vi "HVBuncher.UpdateChannelVoltage.vi"(0 "i ref in":refnum<vi>, 1 "channel":i32, 2 "ChannelVoltages":dbl[](array[numeric]), 3 "ms timeout (10000)":i32=10000, 5 "error in (no error)":errorcluster) -> (14 "i ref out":refnum<vi>, 16 "actVoltage":dbl, 18 "timed out":bool, 19 "error out":errorcluster)   [LabVIEW 2014, in "HVBuncher.lvlib"]
doc: "Gets the voltage from DIM."
uses:
  HVBuncher.lvlib
  CSCore/CSApplicationBaseClasses/PSChannelBase/PSChannelBase.directionType.ctl
  CSCore/CSApplicationBaseClasses/PSChannelBase/PSChannelBase.serviceType.ctl
  CSlibraries/UtilityLib/UtilityLib.valueStatus.ctl
  CSCore/CSApplicationBaseClasses/PSChannelBase/PSChannelBase.lvlib
  CSlibraries/UtilityLib/UtilityLib.lvlib
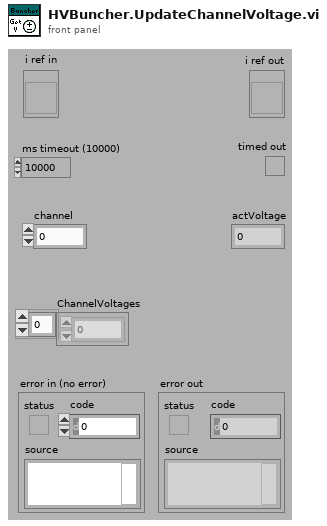
[diagram p1: front panel]
types:
  T1 = typedef "UtilityLib.lvlib/UtilityLib.valueStatus.ctl" = enum16{"no info available", "stand by/off", "on", "warning", "alarm/malfunction", "not implemented", "user action required", "important information", "system default", "control default", "indicator default", "button default"}
  T2 = typedef "PSChannelBase.lvlib/PSChannelBase.serviceType.ctl" = enum16{"onOff", "voltage", "current", "tripCurrent", "rampUpSpeed", "rampDownSpeed", "status"}
  T3 = typedef "PSChannelBase.lvlib/PSChannelBase.directionType.ctl" = enum16{"unknown", "update actual value", "update nominal value", "update both"}
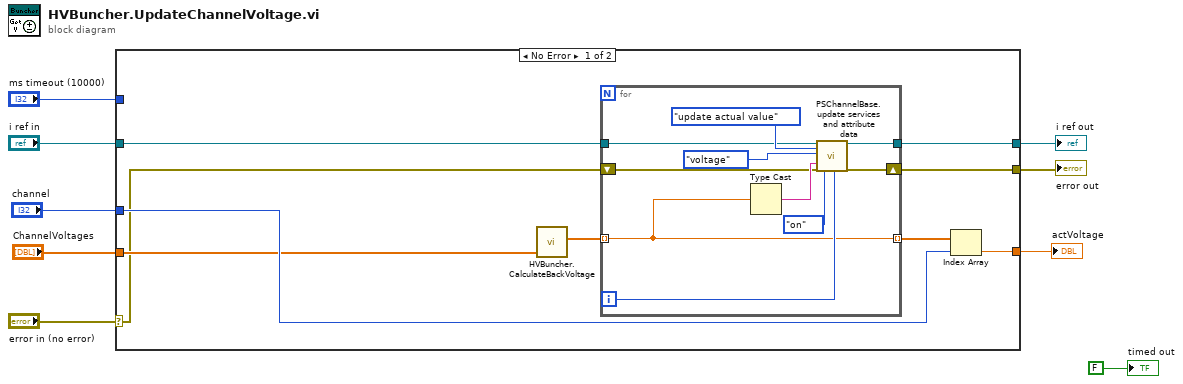
[diagram p0: block diagram]
diagram:
  n1 = case shown="No Error" "error in (no error)" {
    selector: "error in (no error)" -> [w11 w30]
    tunnel: "i ref in" -> [w10 w29]
    tunnel: "ms timeout (10000)" -> [_ _]
    tunnel: "channel" -> [w13 _]
    tunnel: [w15 w30] -> w4
    tunnel: [w16 w29] -> w3
    tunnel: [w17 _] -> w2
    tunnel: "ChannelVoltages" -> [w12 _]
    frame No Error {
      n2 = call "HVBuncher.CalculateBackVoltage.vi"("ChannelVoltages"=w12) -> ("actlVoltages"=w14:dbl[])  [unwired: 10 in]
      n3 = for {
        tunnel: w10 -> [w20]
        shift-right: [w24] -> w15
        shift-left: w11 -> [w21]
        tunnel: [w23] -> w16
        tunnel: [w19] -> w18 mode=indexing
        tunnel: w14 -> [w19] mode=indexing
        i -> [w22]
        n4 = Type Cast(x=w19) -> (*(type *) &x=w26:string)  [unwired: 1 in]
        n5 = call "PSChannelBase.update services and attribute data.vi"("i ref in"=w20, "direction"=PSChannelBase.directionType."update actual value", "service"=PSChannelBase.serviceType."voltage", "value"=w26, "error in (no error)"=w21, "quality"=UtilityLib.valueStatus."on", "channelNumber"=w22) -> ("i ref out"=w23:refnum<vi>, "error out"=w24:errorcluster)  [unwired: 10 in, 1 out]
      }
      n6 = Index Array(array=w18, index=w13) -> (element=w17:dbl)
    }
    frame Error {
    }
  }
  "error out" <- w4
  "i ref out" <- w3
  "actVoltage" <- w2
  "timed out" <- FALSE ("timed out")
